vi "单信号修改.vi"() -> ()   [LabVIEW 2018]
panel:
  in  "修改后控件名称":string
  in  "修改":bool
  in  "修改控件类型":T1(ring)
  in  "修改控件名称":string
  in  "VI路径":path
  in  "GetVIRef":bool
  in  "停止":bool
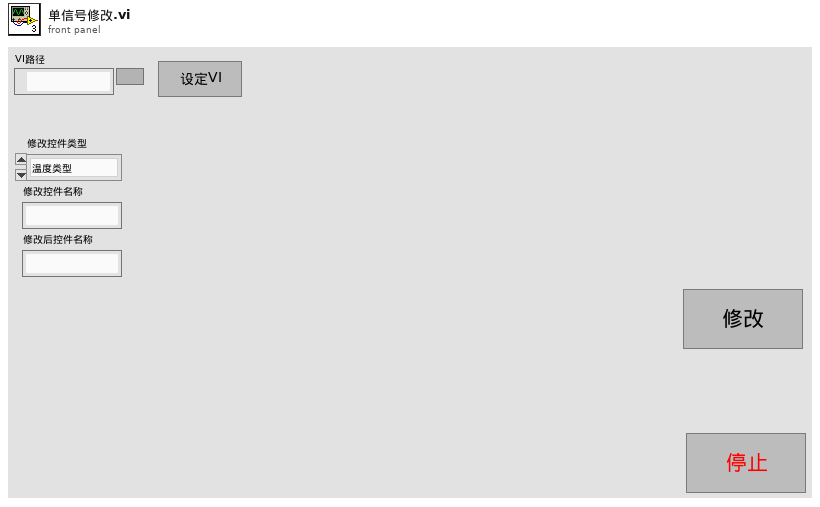
[diagram p1: front panel]
types:
  T1 = enum16{"温度类型", "压力类型", "压差类型", "流量类型", "液位类型", "电流类型", "电压类型", "调节阀", "开关阀"}
  T2 = cluster{"Error":errorcluster, "VI路径":path, "VI引用":refnum<vi>, "退出":bool, "修改控件名称":string, "修改控件类型":enum16{"温度类型", "压力类型", "压差类型", "流量类型", "液位类型", "电流类型", "电压类型", "调节阀", "开关阀"}, "修改后控件名称":string}
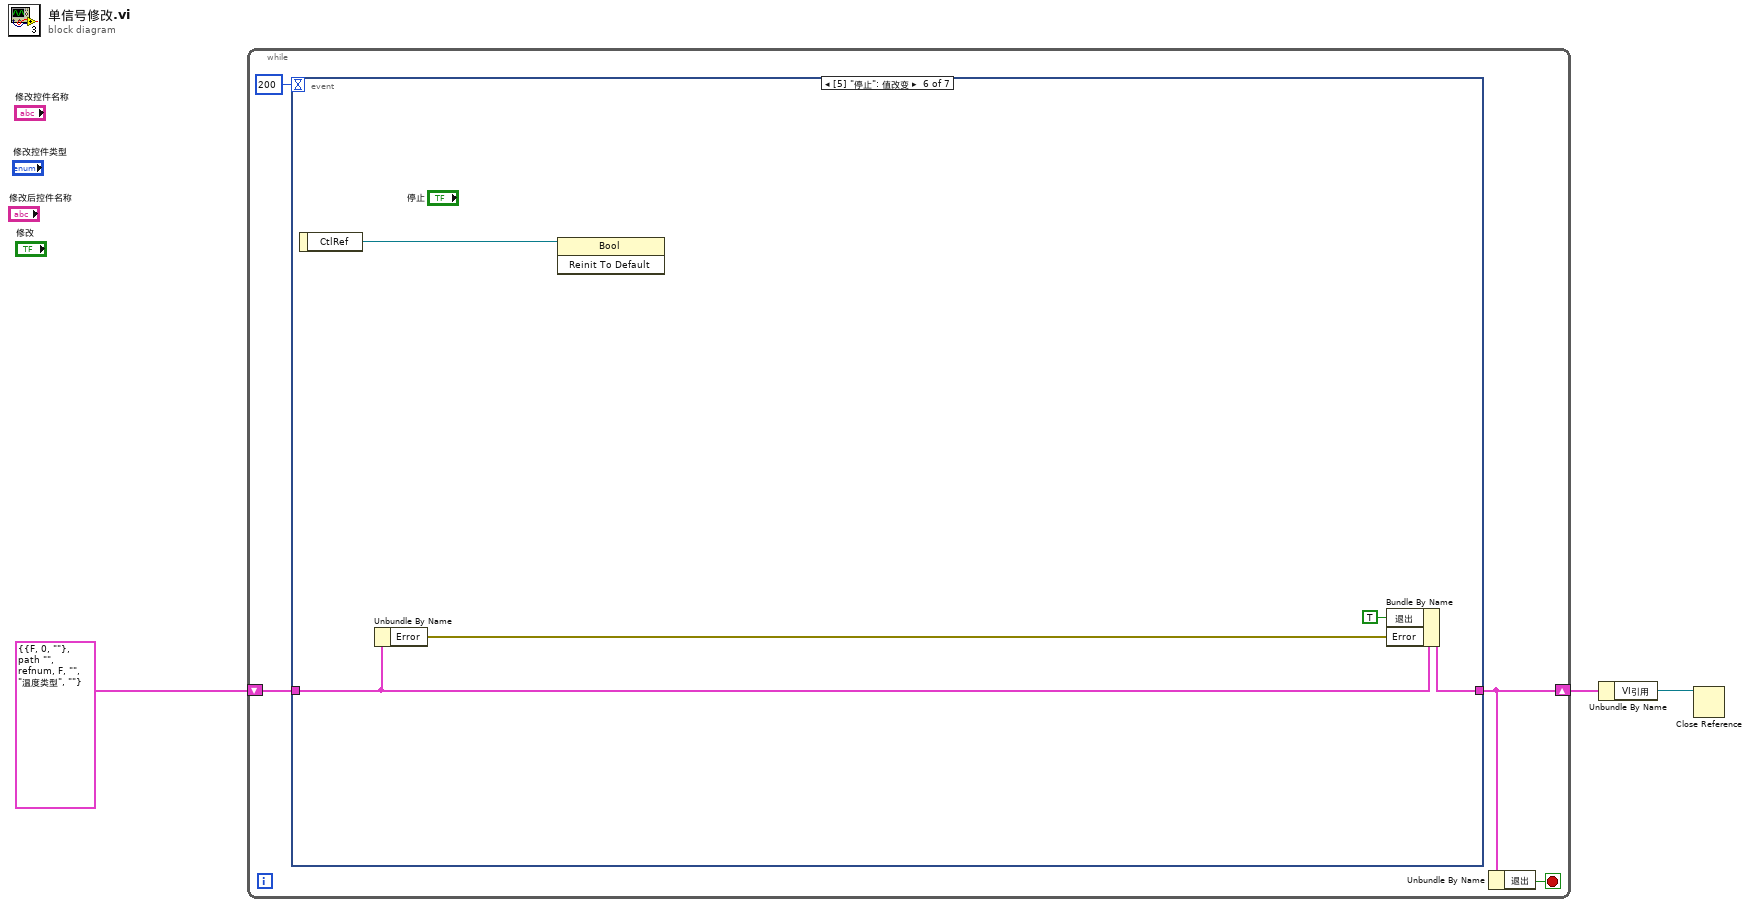
[diagram p0: block diagram]
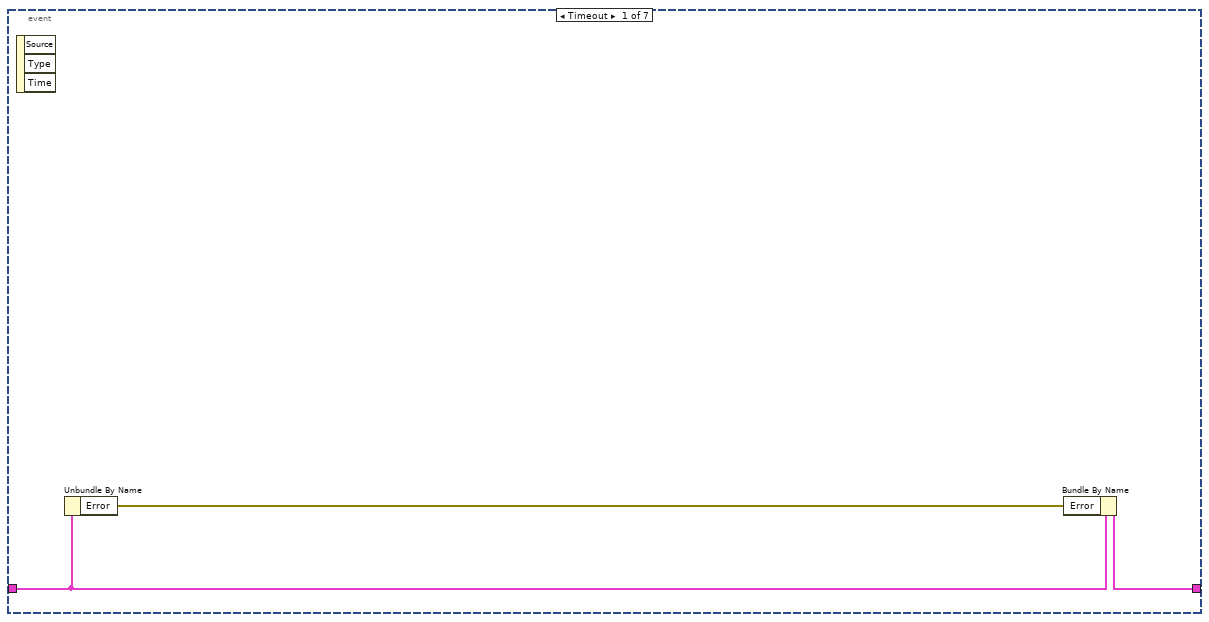
[diagram p2: hidden frame]
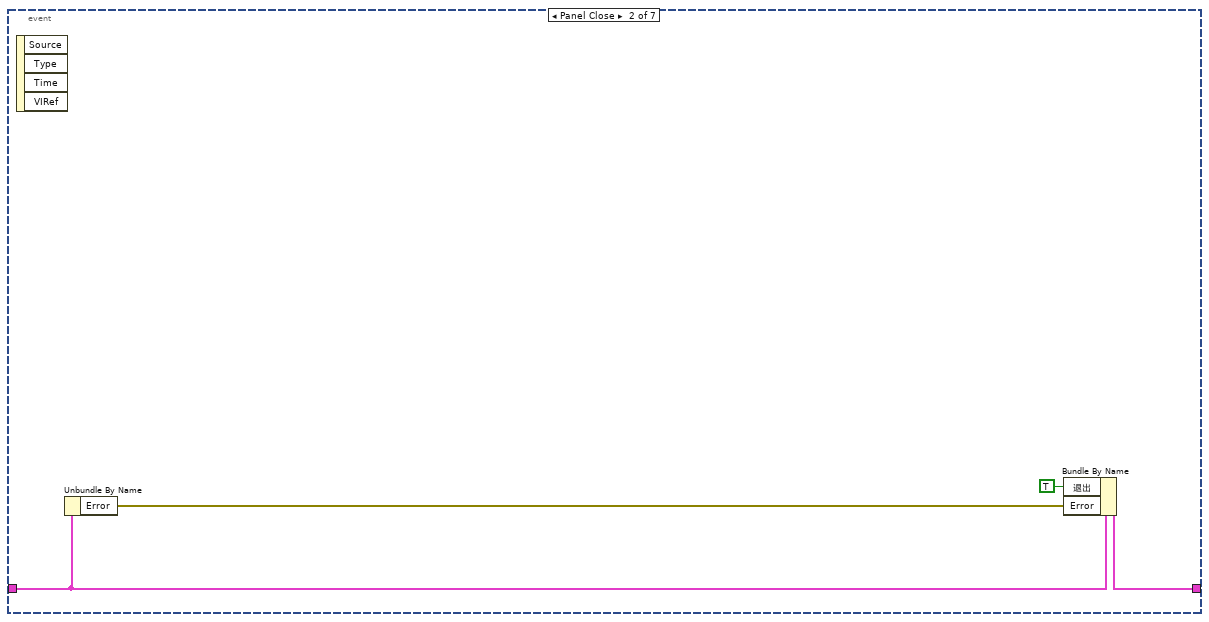
[diagram p3: hidden frame]
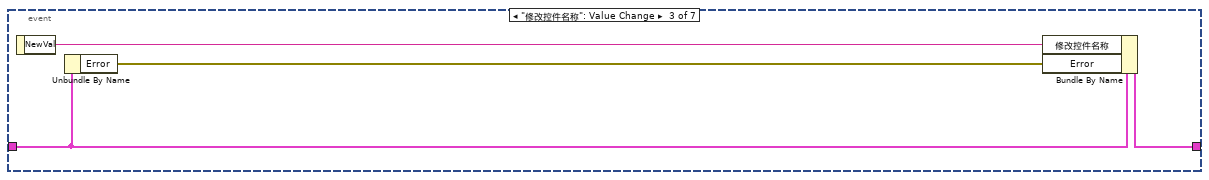
[diagram p4: hidden frame]
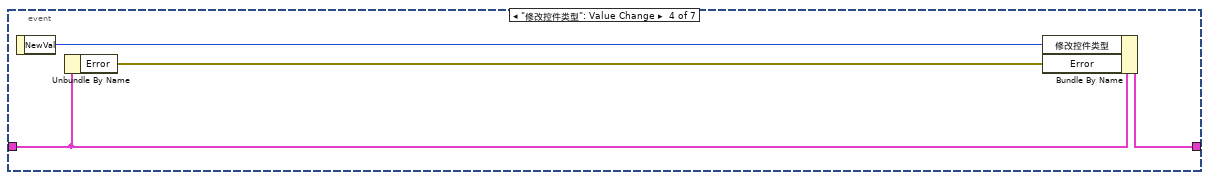
[diagram p5: hidden frame]
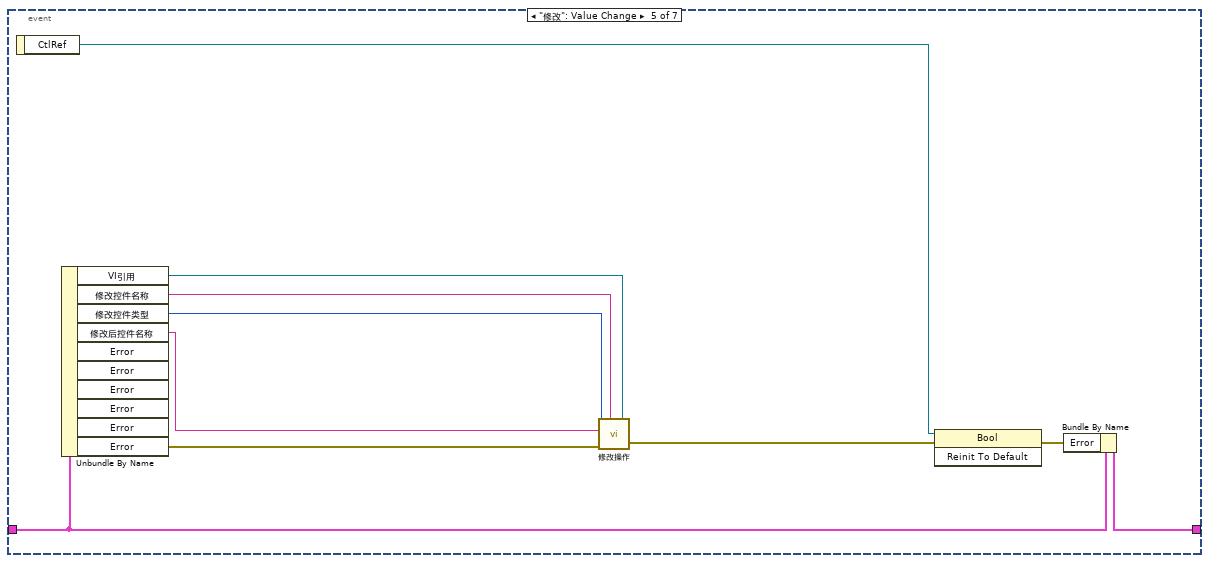
[diagram p6: hidden frame]
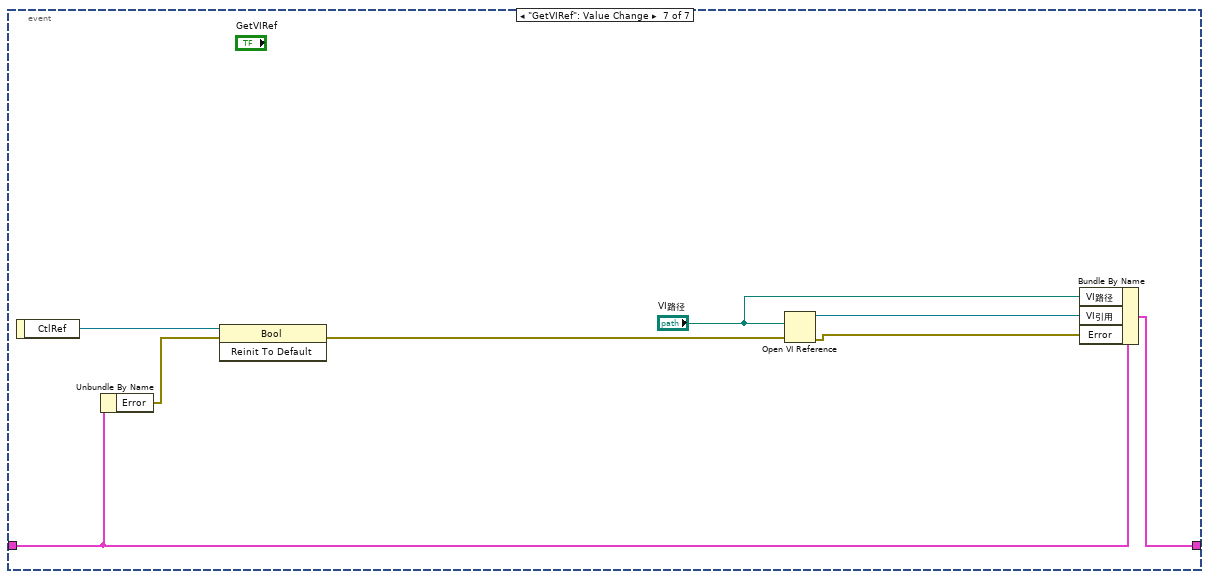
[diagram p7: hidden frame]
diagram:
  n1 = while {
    shift-right: [w5] -> w2
    shift-left: T2 {"Error"={"status"=FALSE, "code"=0, "source"=""}, "VI路径"=path "", "VI引用"=refnum, "退出"=FALSE, "修改控件名称"="", "修改控件类型"=enum."温度类型", "修改后控件名称"=""} -> [w6]
    stop <- w4 stop-if-true
    n2 = event shown="[5] \"停止\": 值改变" {
      selector: _ -> [_ _ _ _ _ _ _]
      dyn-events: _ -> [_ _ _ _ _ _ _]
      timeout: 200 -> [_ _ _ _ _ _ _]
      tunnel: w6 -> [w10 w14 w18 w22 w32 w36 w44]
      tunnel: [w9 w13 w17 w21 w31 w35 w38] -> w5
      event Timeout {
        n3 = event-data() -> ()  [unwired: 1 in, 3 out]
        n4 = Unbundle By Name(w10) -> ("Error"=w8:errorcluster)
        n5 = Bundle By Name(cluster=w10, "Error"=w8) -> (w9:T2)
      }
      event Panel Close {
        n6 = event-data() -> ()  [unwired: 1 in, 4 out]
        n7 = Unbundle By Name(w14) -> ("Error"=w12:errorcluster)
        n8 = Bundle By Name(cluster=w14, "退出"=TRUE, "Error"=w12) -> (w13:T2)
      }
      event "修改控件名称": Value Change {
        n9 = event-data() -> ("NewVal"=w15:string)  [unwired: 1 in]
        n10 = Unbundle By Name(w18) -> ("Error"=w16:errorcluster)
        n11 = Bundle By Name(cluster=w18, "修改控件名称"=w15, "Error"=w16) -> (w17:T2)
      }
      event "修改控件类型": Value Change {
        n12 = event-data() -> ("NewVal"=w19:T1)  [unwired: 1 in]
        n13 = Unbundle By Name(w22) -> ("Error"=w20:errorcluster)
        n14 = Bundle By Name(cluster=w22, "修改控件类型"=w19, "Error"=w20) -> (w21:T2)
      }
      event "修改": Value Change {
        n15 = event-data() -> ("CtlRef"=w30:refnum<vi>)  [unwired: 1 in]
        n16 = Unbundle By Name(w32) -> ("VI引用"=w28:refnum<vi>, "修改控件名称"=w23:string, "修改控件类型"=w27:T1, "修改后控件名称"=w24:string, "Error"=w26:errorcluster)  [unwired: 5 out]
        n17 = call "修改操作.vi"("VI输入"=w28, "修改控件名称"=w23, "错误输入（无错误）"=w26, "修改后控件名称"=w24, "修改控件类型"=w27) -> ("错误输出"=w25:errorcluster)  [unwired: 2 in]
        n18 = invoke class="Bool" method="Reinit To Default"(reference=w30, error in=w25) -> (error out=w29:errorcluster)  [unwired: 1 in, 2 out]
        n19 = Bundle By Name(cluster=w32, "Error"=w29) -> (w31:T2)
      }
      event "停止": Value Change {
        n20 = event-data() -> ("CtlRef"=w37:refnum<vi>)  [unwired: 1 in]
        n21 = Unbundle By Name(w36) -> ("Error"=w34:errorcluster)
        n22 = invoke class="Bool" method="Reinit To Default"(reference=w37) -> ()  [unwired: 2 in, 3 out]
        n23 = Bundle By Name(cluster=w36, "退出"=TRUE ("停止"), "Error"=w34) -> (w35:T2)
      }
      event "GetVIRef": Value Change {
        n24 = event-data() -> ("CtlRef"=w45:refnum<vi>)  [unwired: 1 in]
        n25 = Unbundle By Name(w44) -> ("Error"=w43:errorcluster)
        n26 = invoke class="Bool" method="Reinit To Default"(reference=w45, error in=w43) -> (error out=w42:errorcluster)  [unwired: 1 in, 2 out]
        n27 = Open VI Reference(vi path="VI路径", error in (no error)=w42) -> (vi reference=w41:refnum<vi>, error out=w39:errorcluster)  [unwired: 4 in]
        n28 = Bundle By Name(cluster=w44, "VI路径"="VI路径", "VI引用"=w41, "Error"=w39) -> (w38:T2)
      }
    }
    n29 = Unbundle By Name(w5) -> ("退出"=w4:bool)
  }
  n30 = Unbundle By Name(w2) -> ("VI引用"=w1:refnum<vi>)
  n31 = Close Reference(reference=w1) -> ()  [unwired: 1 in, 1 out]
